vi "TDC_DAQV30_Paralled_muon.vi"(7 "address":string[](array[string])=["192.168.10.20"], 8 "error in (no error)":errorcluster, 9 "stop":bool, 10 "save data":bool=TRUE, 11 "SMA mode":bool=TRUE) -> (0 "error out 3":errorcluster, 2 "csv path":path=path "G:/tdc/2017/data/test_20250313_082908.csv", 3 "rate":dbl)   [LabVIEW 2017]
uses:
  gloabal.vi
  <vilib>/Utility/file.llb/Write Delimited Spreadsheet (DBL).vi
  <vilib>/Utility/file.llb/Write Delimited Spreadsheet (I64).vi
panel:
  out "pmt trigger rate":u32[](array[numeric])
  out "event":u32[](array[numeric])
  in  "calib_file":path=path "G:/tdc/2017/data/test_20250313_032748_codeDensity.csv" caption="文件路径 （空时为对话框）"
  in  "use_calib_file":bool
  out "cal 3":u32[](graph)=[0, 0, 0, 0, 0, 0, 0, 0, 0, 0, 0, 0, 0, 0, 0, 0, 0, 0, 0, 0, 0, 0, 0, 0, 0, 0, 0, 0, 0, 0, 0, 0, 0, 0, 0, 0, 0, 0, 0, 0, 0, 0, 0, 0, 0, 0, 0, 0, 0, 0, 0, 0, 0, 0, 0, 0, 0, 0, 0, 0, 0, 0, 0, 0, 0, 0, 0, 0, 0, 0, 0, 0, 0, 0, 0, 0, 0, 0, 0, 0, 0, 0, 0, 0, 0, 0, 0, 0, 0, 0, 0, 0, 0, 0, 0, 0, 0, 0, 0, 0, 0, 0, 0, 0, 0, 0, 0, 0, 0, 0, 0, 0, 0, 0, 0, 0, 0, 0, 0, 0, 0, 0, 0, 0, 0, 0, 0, 0, 0, 0, 0, 0, 0, 0, 0, 0, 0, 0, 0, 0, 0, 0, 0, 0, 0, 0, 0, 0, 0, 0, 0, 0, 0, 0, 0, 0, 0, 0, 0, 0, 0, 0, 0, 0, 0, 15, 3, 1, 14, 3, 31, 20, 16, 6, 1, 18, 12, 4, 29, 10, 8, 29, 2, 14, 4, 25, 7, 24, 4, 0, 1, 5, 8, 18, 22, 0, 4, 5, 0, 12, 9, 9, 20, 21, 4, 10, 13, 5, 21, 13, 14, 2, 6, 13, 1, 3, 5, 10, 20, 2, 3, 4, 3, 4, 2, 20, 13, 2, 5, 1, 3, 12, 4, 1, 14, 7, 5, 4, 1, 10, 2, 21, 14, 2, 5, 10, 4, 0, 11, 19, 6, 4, 1, 37, 1, 4, 2, 1, 10, 13, 4, 8, 10, 6, 9, 2, 0, 6, 8, 12, 3, 21, 5, 7, 8, 2, 3, 7, 17, 6, 5, 6, 4, 6, 0, 2, 1, 3, 10, 33, 7, 2, 6, 3, 7, 3, 2, 0, 12, 10, 11, 13, 13, 7, 3, 9, 6, 16, 0, 13, 5, 6, 3, 0, 5, 5, 7, 1, 10, 7, 13, 14, 5, 1, 12, 7, 1, 10, 2, 1, 14, 18, 13, 11, 4, 6, 9, 22, 11, 9, 2, 2, 8, 14, 4, 4, 6, 12, 13, 3, 9, 5, 5, 1, 5, 11, 18, 3, 0, 5, 4, 6, 7, 6, 1, 13, 5, 1, 2, 2, 1, 4, 12, 7, 3, 2, 3, 9, 11, 1, 20, 3, 4, 5, 5, 3, 5, 8, 5, 3, 26, 14, 6, 1, 3, 12, 12, 4, 23, 10, 3, 4, 4, 10, 3, 5, 4, 2, 14, 5, 15, 20, 1, 5, 1, 20, 6, 1, 3, 13, 21, 12, 7, 4, 1, 5, 30, 11, 2, 4, 0, 12, 7, 10, 3, 2, 25, 6, 1, 3, 6, 3, 8, 37, 4, 6, 2, 2, 4, 3, 5, 6, 13, 6, 9, 22, 1, 3, 7, 7, 4, 8, 33, 2, 1, 15, 3, 8, 23, 21, 2, 2, 27, 13, 3, 5, 10, 4, 18, 5, 5, 8, 0, 1, 8, 12, 4, 3, 0, 4, 8, 4, 7, 4, 2, 11, 13, 3, 0, 7, 5, 3, 4, 8, 4, 20, 2, 13, 4, 8, 6, 17, 4, 2, 1, 15, 2, 15, 5, 19, 0, 4, 15, 4, 16, 11, 1, 16, 4, 6, 6, 5, 7, 3, 9, 15, 3, 6, 3, 13, 5, 7, 3, 27, 2, 0, 21, 1, 4, 1, 4, 5, 3, 10, 7, 3, 6, 4, 18, 21, 7, 6, 7, 7, 12, 6, 9, 8, 11, 12, 13, 2, 2, 5, 4, 7, 52, 3, 5, 8, 7, 10, 4, 4, 6, 5, 18, 0, 3, 6, 1, 9, 5, 19, 13, 24, 12, 4, 4, 15, 6, 41, 3, 8, 5, 17, 26, 8, 7, 20, 2, 5, 12, 10, 10, 12, 9, 17, 6, 3, 1, 5, 3, 7, 8, 4, 10, 5, 10, 7, 1, 2, 14, 7, 25, 3, 0, 0, 0, 5, 21, 8, 14, 4, 10, 2, 3, 2, 4, 8, 12, 3, 6, 8, 3, 4, 3, 20, 5, 6, 7, 8, 11, 2, 8, 6, 5, 15, 17, 10, 10, 3, 3, 9, 18, 7, 7, 3, 5, 5, 5, 2, 2, 2, 4, 1, 0, 42, 3, 14, 4, 3, 5, 2, 7, 4, 2, 7, 5, 22, 4, 3, 17, 3, 5, 8, 19, 7, 5, 0, 3, 4, 10, 1, 8, 2, 2, 13, 23, 4, 9, 5, 0, 0, 0, 27, 2, 16, 11, 15, 3, 0, 18, 2, 8, 29, 19, 6, 7, 2, 6, 12, 1, 13, 2, 7, 5, 11, 8, 5, 6, 6, 19, 2, 4, 0, 7, 22, 13, 3, 7, 3, 8, 11, 0, 3, 26, 6, 5, 5, 6, 4, 10, 17, 16, 4, 3, 4, 3, 4, 21, 8, 10, 10, 7, 0, 9, 9, 2, 10, 10, 2, 9, 9, 4, 14, 5, 5, 4, 18, 6, 3, 0, 4, 1, 20, 2, 33, 4, 1, 2, 1, 20, 6, 3, 11, 10, 2, 1, 13, 9, 6, 1, 0, 0, 0, 0, 0, 0, 0, 0, 0, 0, 0, 0, 0, 0, 0, 0, 0, 0, 0, 0, 0, 0, 0, 0, 0, 0, 0, 0, 0, 0, 0, 0, 0, 0, 0, 0, 0, 0, 0, 0, 0, 0, 0, 0, 0, 0, 0, 0, 0, 0, 0, 0, 0, 0, 0, 0, 0, 0, 0, 0, 0, 0, 0, 0, 0, 0, 0, 0, 0, 0, 0, 0, 0, 0, 0, 0, 0, 0, 0, 0, 0, 0, 0, 0, 0, 0, 0, 0, 0, 0, 0, 0, 0, 0, 0, 0, 0, 0, 0, 0, 0, 0, 0, 0, 0, 0, 0, 0, 0, 0, 0, 0, 0, 0, 0, 0, 0, 0, 0, 0, 0, 0, 0, 0, 0, 0, 0, 0, 0, 0, 0, 0, 0, 0, 0, 0, 0, 0, 0, 0, 0, 0, 0, 0, 0, 0, 0, 0, 0, 0, 0, 0, 0, 0, 0, 0, 0, 0, 0, 0, 0, 0, 0, 0, 0, 0, 0, 0, 0, 0, 0, 0, 0, 0, 0, 0, 0, 0, 0, 0, 0, 0, 0, 0, 0, 0, 0, 0, 0, 0, 0, 0, 0, 0, 0, 0, 0, 0, 0, 0, 0, 0, 0, 0, 0, 0, 0, 0, 0, 0, 0, 0, 0, 0, 0, 0, 0, 0, 0, 0, 0, 0, 0, 0, 0, 0, 0, 0, 0, 0, 0, 0, 0, 0, 0, 0, 0, 0, 0, 0, 0, 0, 0, 0, 0, 0, 0, 0, 0, 0, 0, 0, 0, 0, 0, 0, 0, 0, 0, 0, 0, 0, 0, 0, 0, 0, 0, 0, 0, 0, 0, 0, 0, 0, 0, 0, 0, 0, 0, 0, 0, 0, 0, 0, 0, 0, 0, 0, 0, 0, 0, 0, 0, 0, 0, 0, 0, 0, 0, 0, 0, 0, 0, 0, 0, 0, 0, 0, 0, 0, 0, 0, 0, 0, 0, 0, 0, 0, 0, 0, 0, 0, 0, 0, 0, 0, 0, 0, 0, 0, 0, 0, 0, 0, 0, 0, 0, 0, 0, 0, 0, 0, 0, 0, 0, 0, 0, 0, 0, 0, 0, 0, 0, 0, 0, 0, 0, 0, 0, 0, 0, 0, 0, 0, 0, 0, 0, 0, 0, 0, 0, 0, 0, 0, 0, 0, 0, 0, 0, 0, 0, 0, 0, 0, 0, 0, 0, 0, 0, 0, 0, 0, 0, 0, 0, 0, 0, 0, 0, 0, 0, 0, 0, 0, 0, 0, 0, 0, 0, 0, 0, 0, 0, 0, 0, 0, 0, 0, 0, 0, 0, 0, 0, 0, 0, 0, 0, 0, 0, 0, 0, 0, 0, 0, 0, 0, 0, 0, 0, 0, 0, 0, 0, 0, 0, 0, 0, 0, 0, 0, 0, 0, 0, 0, 0, 0, 0, 0, 0, 0, 0, 0, 0, 0, 0, 0, 0, 0, 0, 0, 0, 0, 0, 0, 0, 0, 0, 0, 0, 0, 0, 0, 0, 0, 0, 0, 0, 0, 0, 0, 0, 0, 0, 0, 0, 0, 0, 0, 0, 0, 0, 0, 0, 0, 0, 0, 0, 0, 0, 0, 0, 0, 0, 0, 0, 0, 0, 0, 0, 0, 0, 0, 0, 0, 0, 0, 0, 0, 0, 0, 0, 0, 0, 0, 0, 0, 0, 0, 0, 0, 0, 0, 0, 0, 0, 0, 0, 0, 0, 0, 0, 0, 0, 0, 0, 0, 0, 0, 0, 0, 0, 0, 0, 0, 0, 0, 0, 0, 0, 0, 0, 0, 0, 0, 0, 0, 0, 0, 0, 0, 0, 0, 0, 0, 0, 0, 0, 0, 0, 0, 0, 0, 0, 0, 0, 0, 0, 0, 0, 0, 0, 0, 0, 0, 0, 0, 0, 0, 0, 0, 0, 0, 0, 0, 0, 0, 0, 0, 0, 0, 0, 0, 0, 0, 0, 0, 0, 0, 0, 0, 0, 0, 0, 0, 0, 0, 0, 0, 0, 0, 0, 0, 0, 0, 0, 0, 0, 0, 0, 0, 0, 0, 0, 0, 0, 0, 0, 0, 0, 0, 0, 0, 0, 0, 0, 0, 0, 0, 0, 0, 0, 0, 0, 0, 0, 0, 0, 0, 0, 0, 0, 0, 0, 0, 0, 0, 0, 0, 0, 0, 0, 0, 0, 0, 0, 0, 0, 0, 0, 0, 0, 0, 0, 0, 0, 0, 0, 0, 0, 0, 0, 0, 0, 0, 0, 0, 0, 0, 0, 0, 0, 0, 0, 0, 0, 0, 0, 0, 0, 0, 0, 0, 0, 0, 0, 0, 0, 0, 0, 0, 0, 0, 0, 0, 0, 0, 0, 0, 0, 0, 0, 0, 0, 0, 0, 0, 0, 0, 0, 0, 0, 0, 0, 0, 0, 0, 0, 0, 0, 0, 0, 0, 0, 0, 0, 0, 0, 0, 0, 0, 0, 0, 0, 0, 0, 0, 0, 0, 0, 0, 0, 0, 0, 0, 0, 0, 0, 0, 0, 0, 0, 0, 0, 0, 0, 0, 0, 0, 0, 0, 0, 0, 0, 0, 0, 0, 0, 0, 0, 0, 0, 0, 0, 0, 0, 0, 0, 0, 0, 0, 0, 0, 0, 0, 0, 0, 0, 0, 0, 0, 0, 0, 0, 0, 0, 0, 0, 0, 0, 0, 0, 0, 0, 0, 0, 0, 0, 0, 0, 0, 0, 0, 0, 0, 0, 0, 0, 0, 0, 0, 0, 0, 0, 0, 0, 0, 0, 0, 0, 0, 0, 0, 0, 0, 0, 0, 0, 0, 0, 0, 0, 0, 0, 0, 0, 0, 0, 0, 0, 0, 0, 0, 0, 0, 0, 0, 0, 0, 0, 0, 0, 0, 0, 0, 0, 0, 0, 0, 0, 0, 0, 0, 0, 0, 0, 0, 0, 0, 0, 0, 0, 0, 0, 0, 0, 0, 0, 0, 0, 0, 0, 0, 0, 0, 0, 0, 0, 0, 0, 0, 0, 0, 0, 0, 0, 0, 0, 0, 0, 0, 0, 0, 0, 0, 0, 0, 0, 0, 0, 0, 0, 0, 0, 0, 0, 0, 0, 0, 0, 0, 0, 0, 0, 0, 0, 0, 0, 0, 0, 0, 0, 0, 0, 0, 0, 0, 0, 0, 0, 0, 0, 0, 0, 0, 0, 0, 0, 0, 0, 0, 0, 0, 0, 0, 0, 0, 0, 0, 0, 0, 0, 0, 0, 0, 0, 0, 0, 0, 0, 0, 0, 0, 0, 0, 0, 0, 0, 0, 0, 0, 0, 0, 0, 0, 0, 0, 0, 0, 0, 0, 0, 0, 0, 0, 0, 0, 0, 0, 0, 0, 0, 0, 0, 0, 0, 0, 0, 0, 0, 0, 0, 0, 0, 0, 0, 0, 0, 0, 0, 0, 0, 0, 0, 0, 0, 0, 0, 0, 0, 0, 0, 0, 0, 0, 0, 0, 0, 0, 0, 0, 0, 0, 0, 0, 0, 0, 0, 0, 0, 0, 0, 0, 0, 0, 0, 0, 0, 0, 0, 0, 0, 0, 0, 0, 0, 0, 0, 0, 0, 0, 0, 0, 0, 0, 0, 0, 0, 0, 0, 0, 0, 0, 0, 0, 0, 0, 0, 0, 0, 0, 0, 0, 0, 0, 0, 0, 0, 0, 0, 0, 0, 0, 0, 0, 0, 0, 0, 0, 0, 0, 0, 0, 0, 0, 0, 0, 0, 0, 0, 0, 0, 0, 0, 0, 0, 0, 0, 0, 0, 0, 0, 0, 0, 0, 0, 0, 0, 0, 0, 0, 0, 0, 0, 0, 0, 0, 0, 0, 0, 0, 0, 0, 0, 0, 0, 0, 0, 0, 0, 0, 0, 0, 0, 0, 0]
  out "second stamp":u64=57608
  in  "coarse counter width":u16(ring) items=["29", "48"]
  out "name (unnamed)":string
  out "error out 5":errorcluster
  in  "timeout":dbl=30000.0
  out "DAC":dbl=8094.0
  out "Out":u8=3 format="%.0x"
  out "fine 4":u64=133527214080 format="%x"
  out "coarse":u64=65198835 format="%x"
  in  "gps":bool
  out "Year":string="2025"
  in  "factor":i32=128
  in  "displayCR":bool=TRUE
  in  "Counter Setting":dbl=100000.0 format="%#_13g"
  in  "replace dat":bool
  in  "append csv":bool=TRUE
  out "element":string
  out "fine":u64=593 format="%x"
  in  "UDP Config":bool=TRUE
  in  "data  path":path=path "G:/tdc/2017/data"
  out "cal 2":u64[](graph)
  in  "Thresholds (mV)":dbl[](array[numeric])=[580.0, 580.0, 580.0, 580.0, 600.0, 600.0, 600.0, 600.0, 580.0, 580.0, 600.0, 600.0, 600.0, 600.0, 600.0, 600.0, 580.0, 580.0, 600.0, 600.0, 600.0, 600.0, 600.0, 600.0, 580.0, 580.0, 600.0, 600.0, 600.0, 600.0, 600.0, 600.0, 600.0, 600.0, 600.0, 600.0, 600.0, 600.0, 600.0, 600.0, 600.0, 600.0, 600.0, 600.0, 600.0, 600.0, 600.0, 600.0, 600.0, 600.0, 600.0, 600.0, 600.0, 600.0, 600.0, 600.0, 600.0, 600.0, 600.0, 600.0, 600.0, 600.0, 600.0, 600.0]
  out "error out 2":errorcluster
  in  "display":bool=TRUE
  in  "Thresholds":dbl=-0.03
  in  "one key for threshold":bool=TRUE
  in  "RST":bool
  in  "通道数量":i32=128
  out "Cal Table":u32[](array[numeric])
  in  "channel for cal":i32=3
  out "channel number":u64
  out "Calibration Counter":i32=100000
  out "Event index":i32=97959
  out "cal":i64[](graph)
  out "error out":errorcluster
  out "appended path":path=path "G:/tdc/2017/data/test_20250313_082908.dat"
  in  "filename":string="test"
  in  "Events":i32=110000 min=1
  in  "timeout (ms)":i32=10000
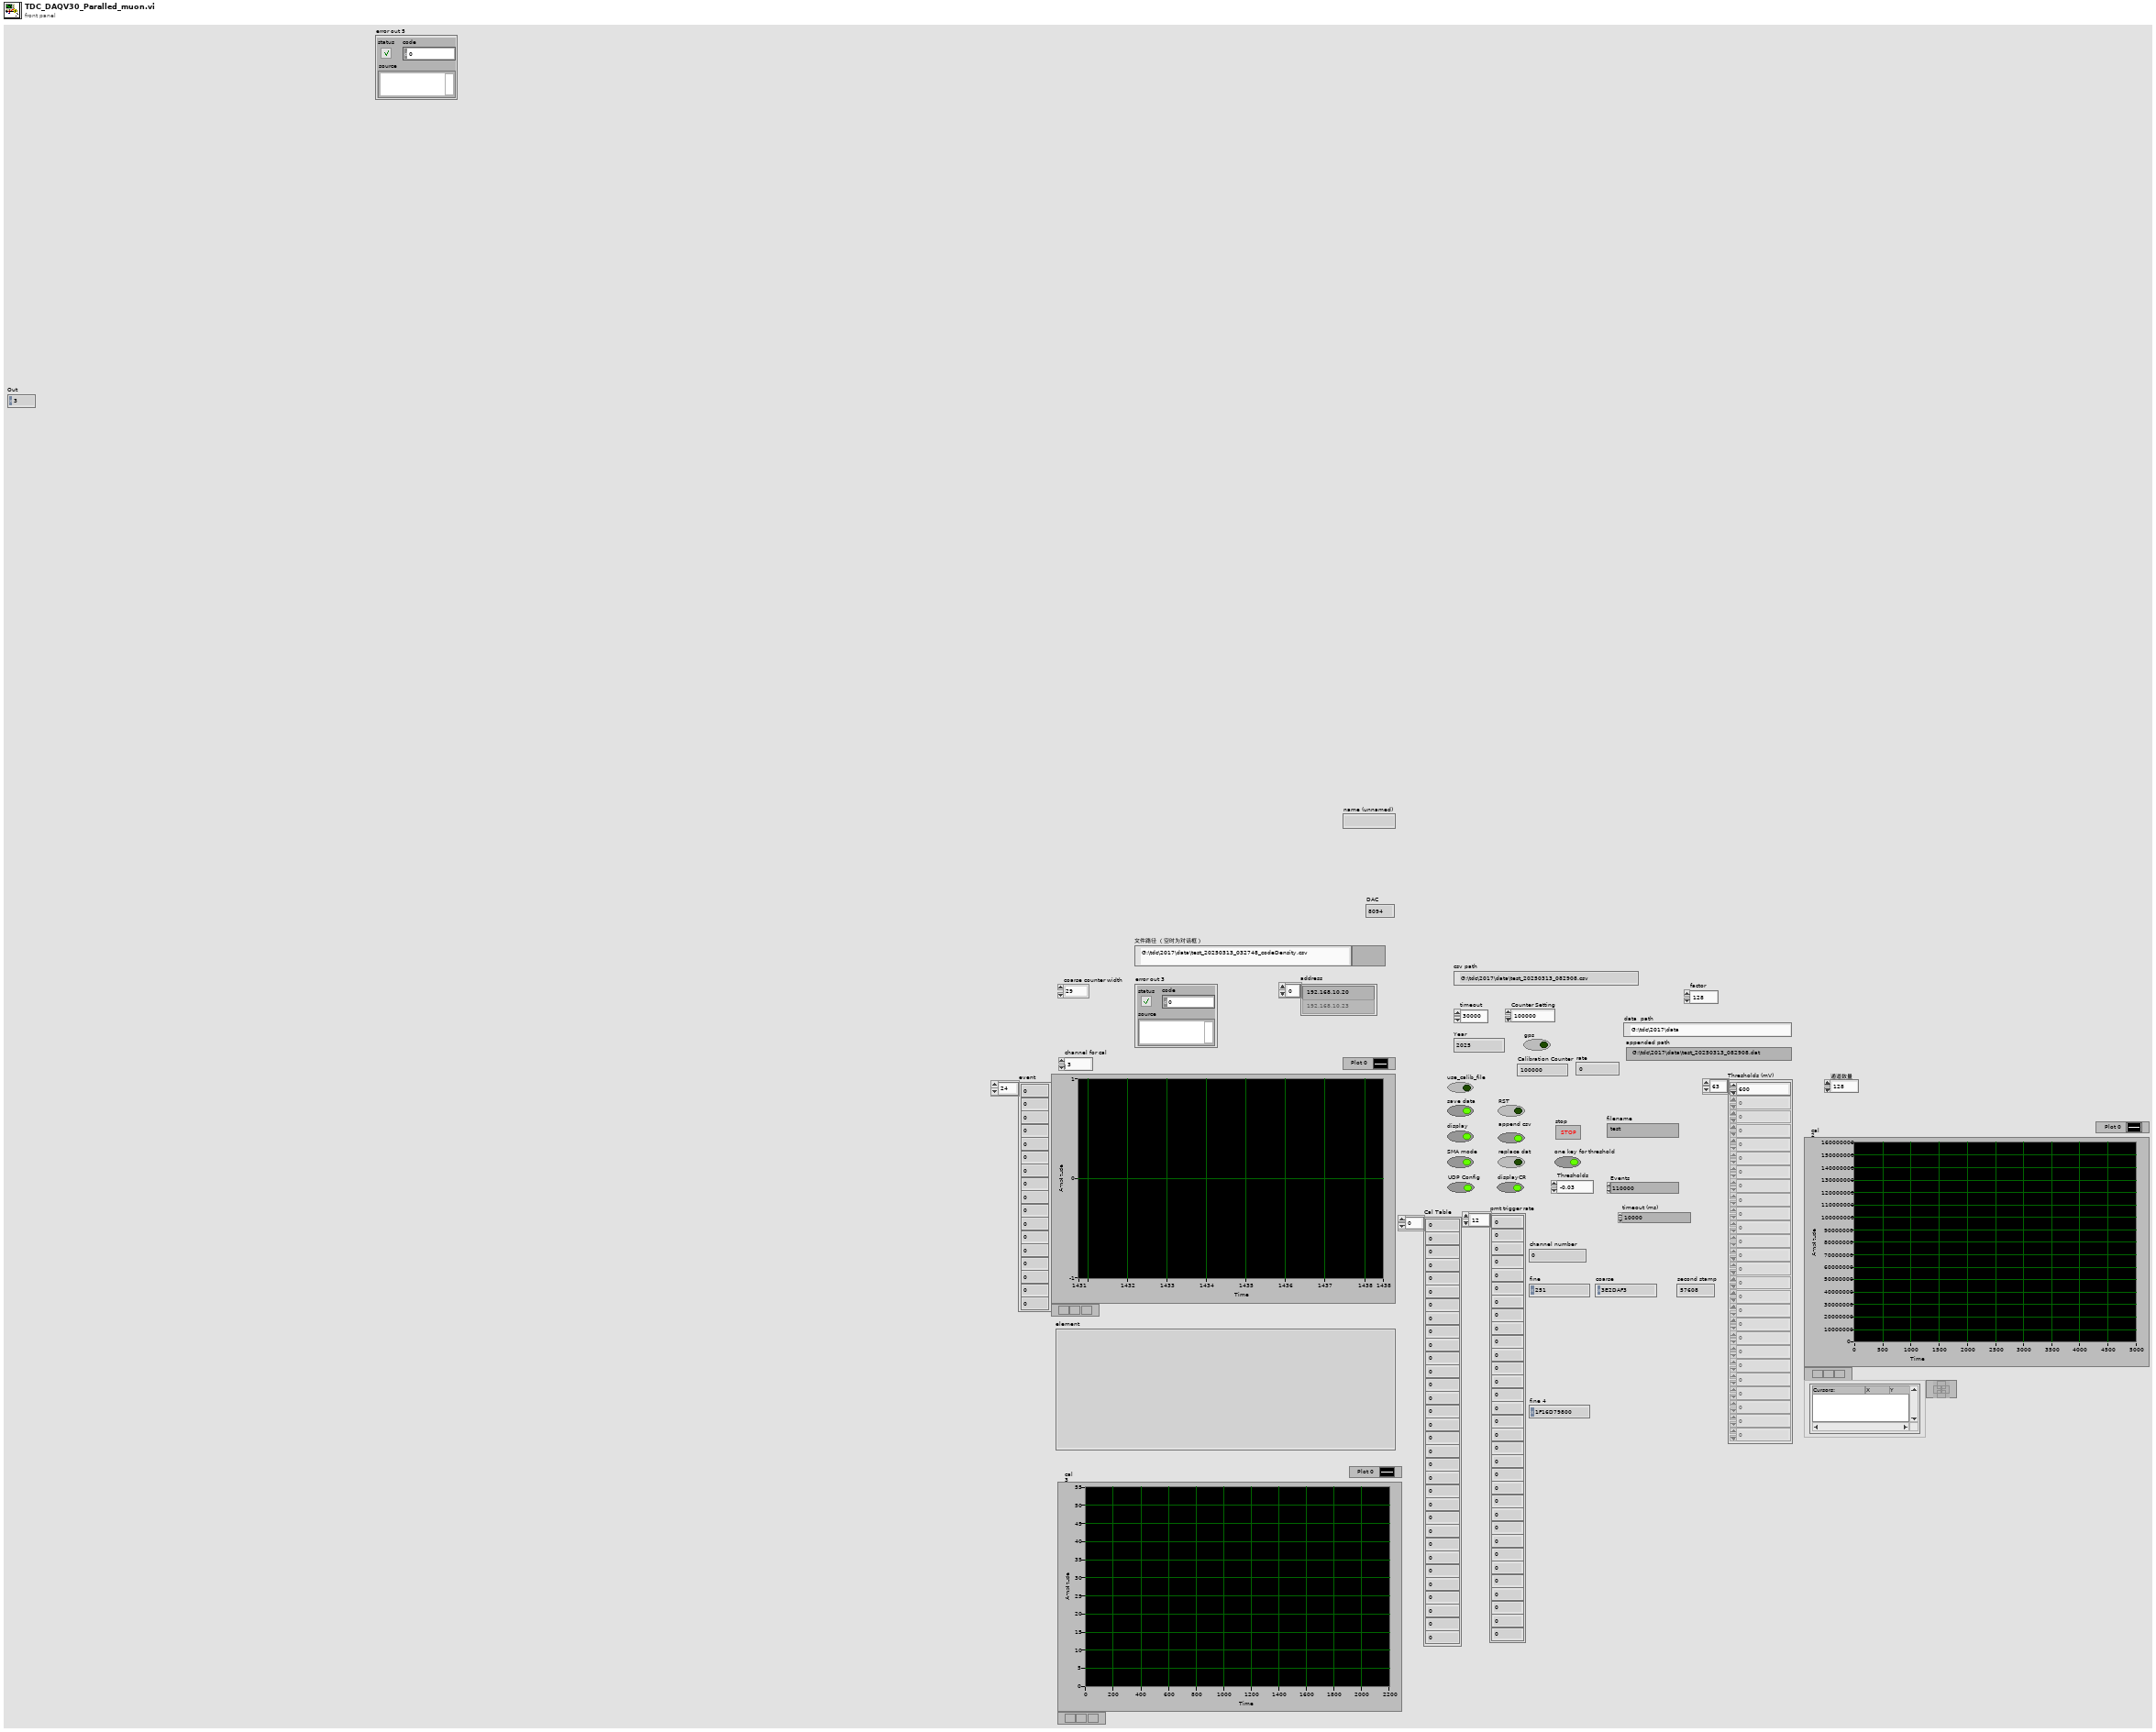
[diagram p1: front panel]
types:
  T1 = enum16{"open", "replace", "create", "open or create", "replace or create", "replace or create with confirmation"}
  T2 = enum16{"big-endian, network order", "native, host order", "little-endian"}
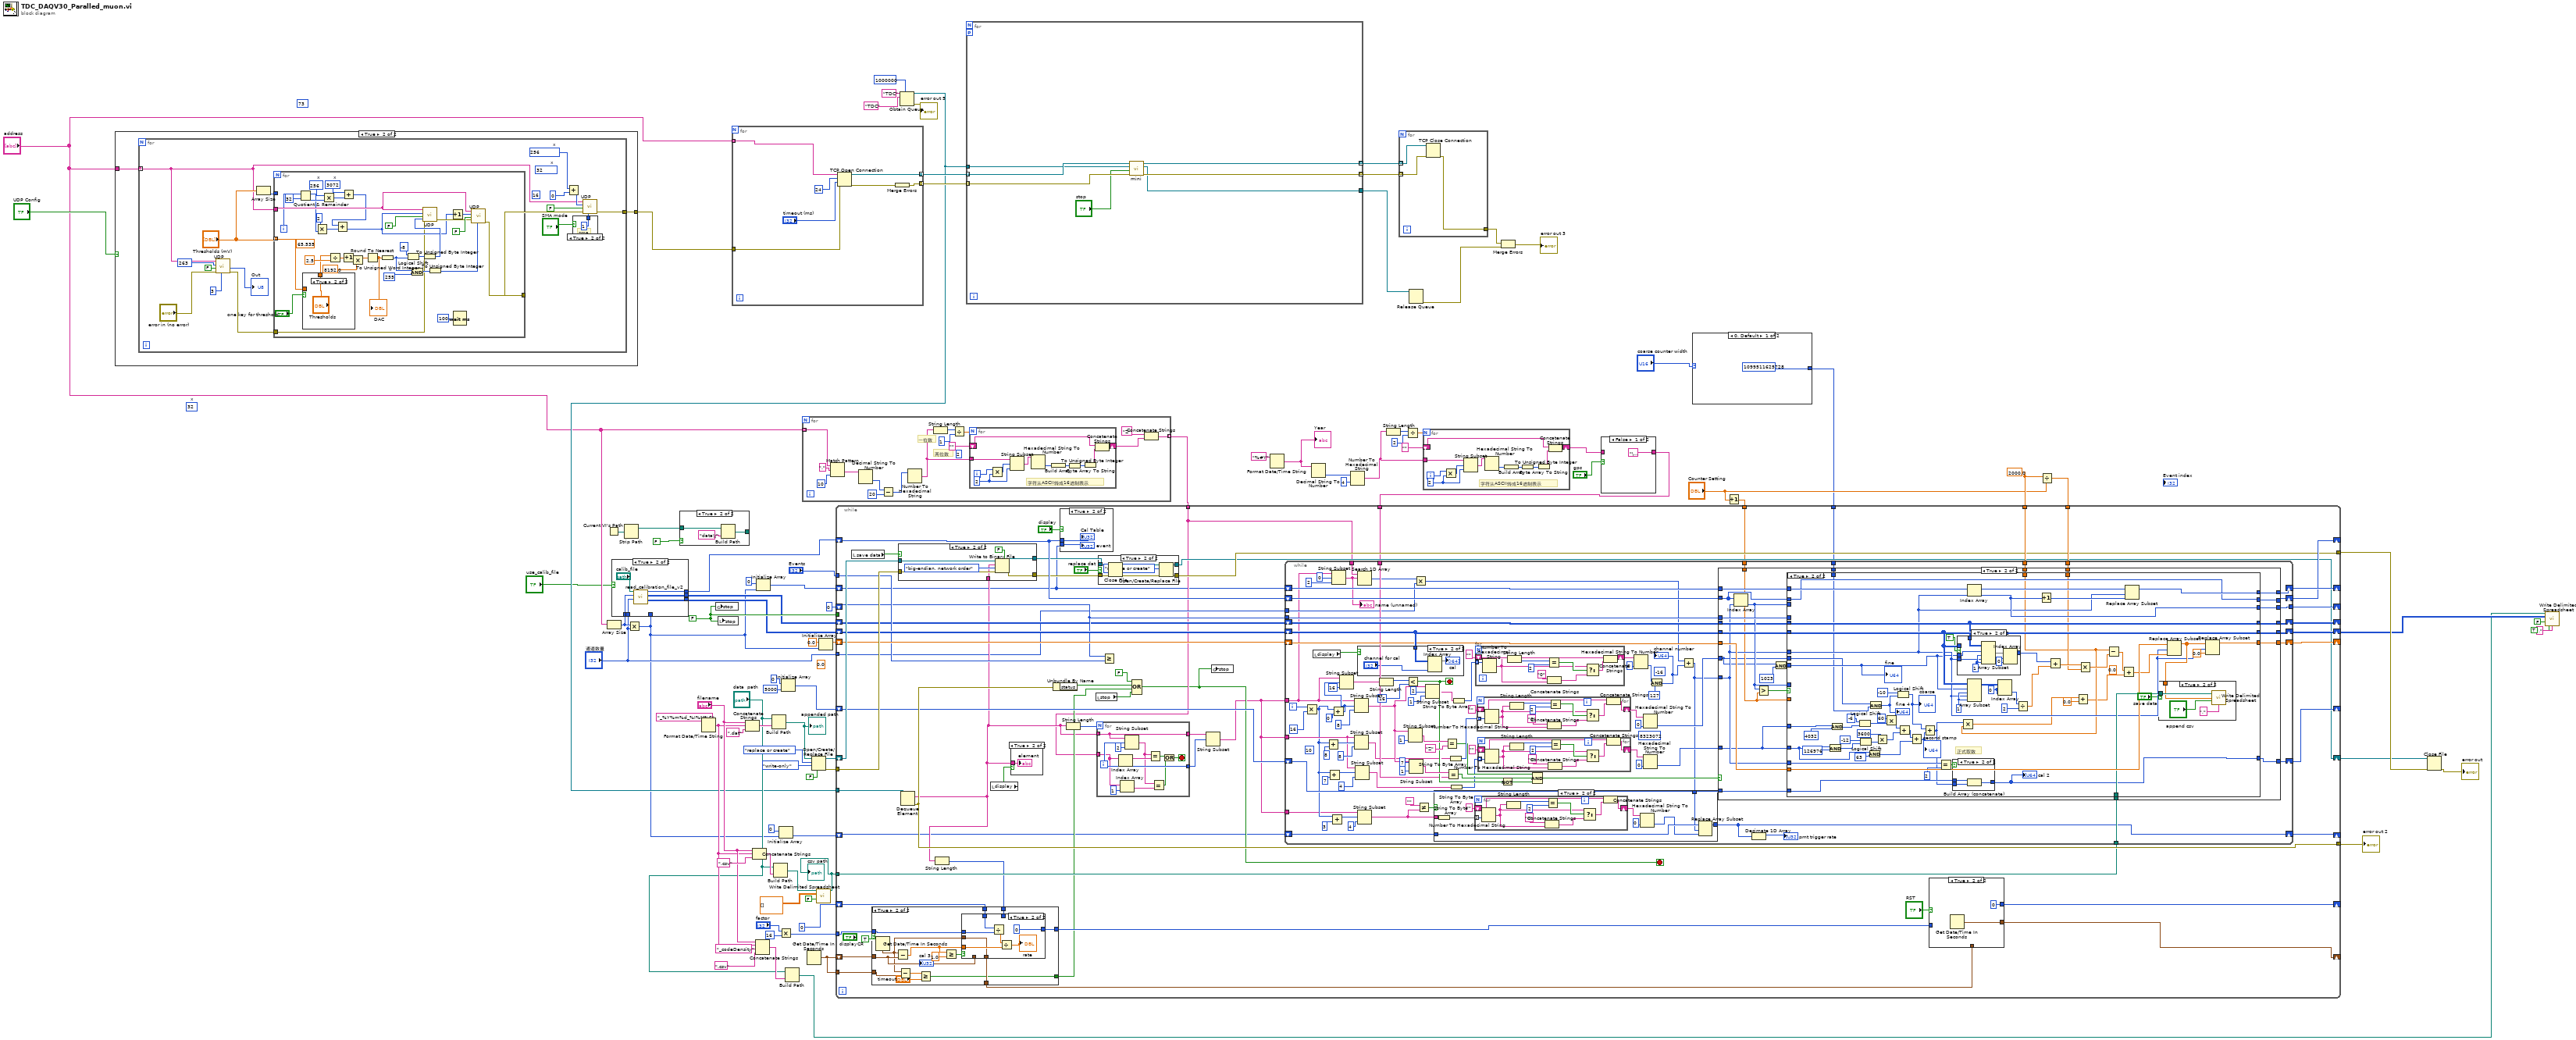
[diagram p0: block diagram]
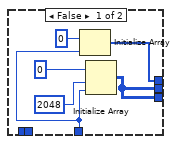
[diagram p2: hidden frame]
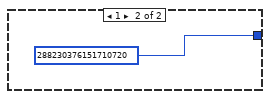
[diagram p3: hidden frame]
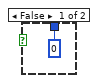
[diagram p6: hidden frame]
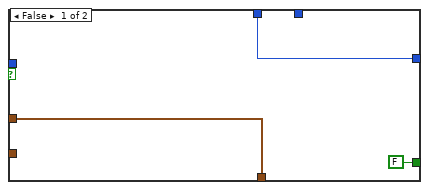
[diagram p12: hidden frame]
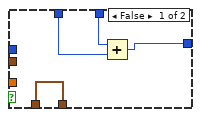
[diagram p13: hidden frame]
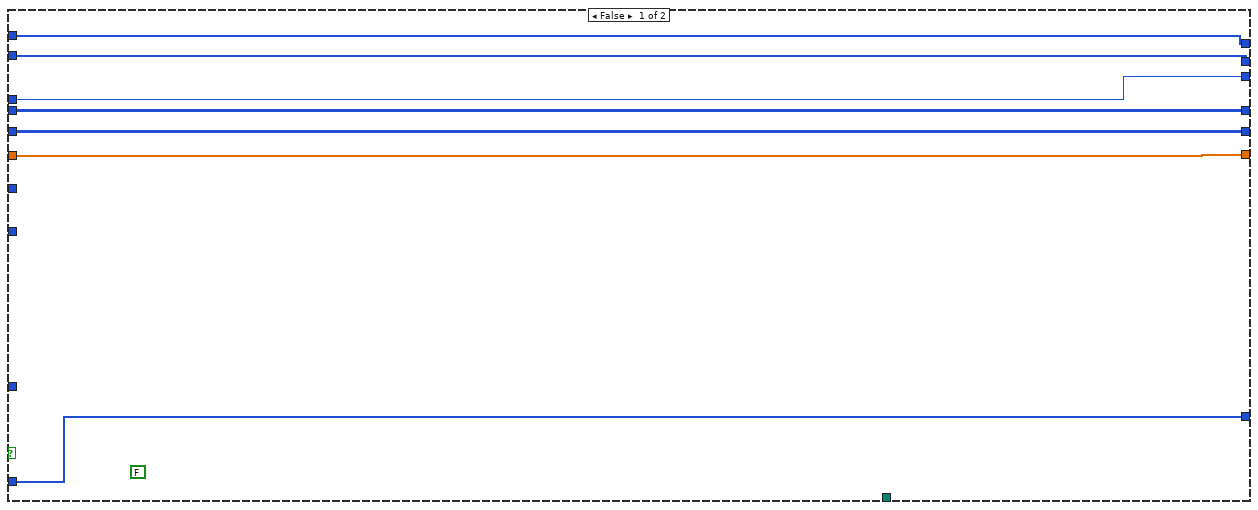
[diagram p18: hidden frame]
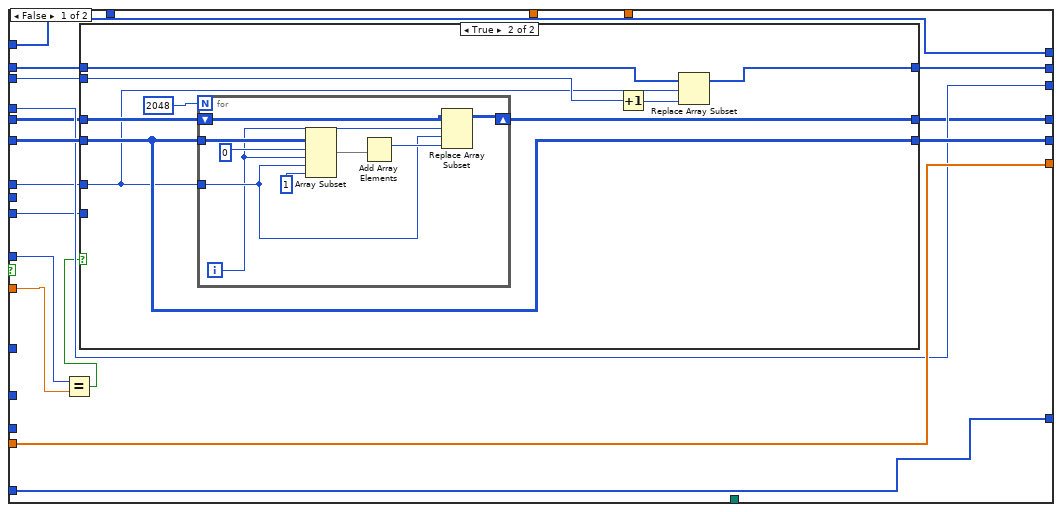
[diagram p19: hidden frame]
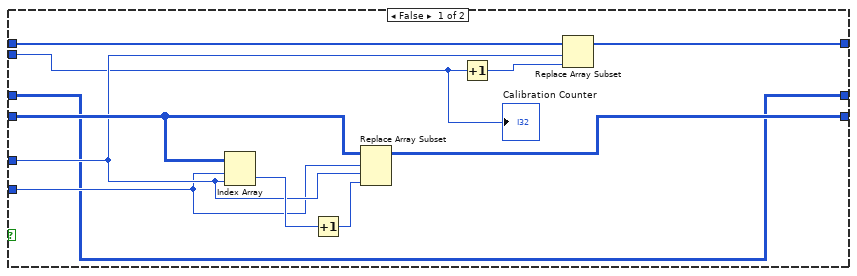
[diagram p20: hidden frame]
diagram:
  (unwired) u32 73 ("Address")
  w51 = 2000.0 ("x")
  (unwired) u16 32  # x
  w13 = FALSE ("stop")
  (unwired) 0.0
  n1 = case shown="True" "UDP Config" {
    tunnel: "address" -> [_ w93]
    tunnel: [_ w94] -> w18
    frame False {
    }
    frame True {
      n2 = for {
        tunnel: [w109] -> w94
        tunnel: w93 -> [w97] mode=indexing
        (unwired) u16 32  # x
        (unwired) u32 16 ("Address")
        w102 = u16 256  # x
        n3 = call "UDP.vi"("In"=u8 3, "error in (no error)"="error in (no error)", "Read (TRUE)"=FALSE, "Address"=u32 263, "IP address"=w97) -> ("error out"=w95:errorcluster, "Out"=→"Out":u8)  [unwired: 3 in, 1 out]
        n4 = Array Size(array="Thresholds (mV)") -> (size(s)=w106:i32)
        n5 = for {
          tunnel: w97 -> [w143]
          tunnel: "Thresholds (mV)" -> [w130] mode=indexing
          tunnel: [w133] -> w110
          tunnel: w106 -> [_]
          tunnel: w95 -> [w117]
          i -> [w125]
          (unwired) 65.535 ("y")
          w126 = u16 3072  # x
          w127 = u16 256  # x
          w139 = u16 255  # x
          n6 = Quotient & Remainder(x=w125, y=32) -> (x-y*floor(x/y)=w119:i32, floor(x/y)=w128:i32)
          n7 = case shown="True" "one key for threshold" {
            tunnel: [w149 "Thresholds"] -> w131
            tunnel: w130 -> [w149 _]
            frame False {
            }
            frame True {
            }
          }
          n8 = Multiply(x=2, y=w119) -> (x*y=w120:i32)
          n9 = Multiply(x=w127, y=w128) -> (x*y=w122:i32)
          n10 = Divide(x=w131, y=2.5) -> (x/y=w146:dbl)
          n11 = Increment(x=w146) -> (x+1=w116:dbl)
          n12 = Add(x=w126, y=w122) -> (x+y=w121:i32)
          n13 = Add(x=w121, y=w120) -> (x+y=w124:i32)
          n14 = Multiply(x=w116, y=8192.0) -> (x*y=w115:dbl)
          n15 = Round To Nearest(number=w115) -> (nearest integer value=w144:dbl)
          "DAC" <- w144
          n16 = To Unsigned Word Integer(number=w144) -> (unsigned 16bit integer=w135:u16)
          n17 = Logical Shift(y=i16 -8, x=w135) -> (x << y=w141:u16)
          n18 = And(x=w135, y=w139) -> (x .and. y?=w138:u16)
          n19 = To Unsigned Byte Integer(number=w141) -> (unsigned 8bit integer=w140:u8)
          n20 = call "UDP.vi"("In"=w140, "error in (no error)"=w117, "Read (TRUE)"=FALSE, "Address"=w124, "IP address"=w143) -> ("error out"=w134:errorcluster)  [unwired: 3 in, 2 out]
          n21 = To Unsigned Byte Integer(number=w138) -> (unsigned 8bit integer=w137:u8)
          n22 = Increment(x=w124) -> (x+1=w123:i32)
          n23 = Wait (ms)(milliseconds to wait=u32 100) -> ()  [unwired: 1 out]
          n24 = call "UDP.vi"("In"=w137, "error in (no error)"=w134, "Read (TRUE)"=FALSE, "Address"=w123, "IP address"=w143) -> ("error out"=w133:errorcluster)  [unwired: 3 in, 2 out]
        }
        n25 = Add(x=w102, y=u32 0 ("Address")) -> (x+y=w103:u32)
        n26 = case shown="True" "SMA mode" {
          tunnel: [u8 0 ("In") u8 1 ("In")] -> w108
          frame False {
          }
          frame True {
            # "sma"
          }
        }
        n27 = call "UDP.vi"("In"=w108, "error in (no error)"=w110, "Read (TRUE)"=FALSE, "Address"=w103, "IP address"=w97) -> ("error out"=w109:errorcluster)  [unwired: 3 in, 2 out]
      }
    }
  }
  n28 = Current VI's Path() -> (path=w87:path)
  n29 = Array Size(array="address") -> (size(s)=w5:i32)
  n30 = Strip Path(path=w87) -> (stripped path=w86:path)  [unwired: 1 out]
  n31 = Multiply(x=w5, y="通道数量") -> (x*y=w2:i32)
  n32 = case shown="True" "use_calib_file" {
    tunnel: w2 -> [w154 _]
    tunnel: [w151 w162] -> w8
    tunnel: [w151 w161] -> w7
    tunnel: [w152 w160] -> w6
    tunnel: w5 -> [_ w159]
    tunnel: "通道数量" -> [_ w158]
    frame False {
      n33 = Initialize Array(u32 0 ("element"), w154) -> (w152:u32[])
      n34 = Initialize Array(u32 0 ("element"), 2048 ("dimension size"), w154) -> (w151:u32[][])
    }
    frame True {
      n35 = call "read_calibration_file_v2.vi"("通道数量"=w158, "板子数量"=w159, "file path (dialog if empty)"="calib_file") -> ("code_density"=w162:i64[][], "accumulation"=w161:u32[][], "Cal Table"=w160:u32[])  [unwired: 5 in, 1 out]
    }
  }
  n36 = case shown="True" FALSE {
    tunnel: w86 -> [w163 w165]
    tunnel: [w163 w164] -> _
    frame False {
    }
    frame True {
      n37 = Build Path(base path=w165, name or relative path="data\\") -> (appended path=w164:path)
    }
  }
  n38 = Format Date/Time String(time format string (%c)="_%Y%m%d_%I%M%S") -> (date/time string=w68:string)  [unwired: 2 in]
  n39 = global write "gloabal.vi" "stop"(w13) -> ()
  n40 = local write "stop"(w13) -> ()
  n41 = for {
    tunnel: "address" -> [w172] mode=indexing
    tunnel: [w171] -> w28 mode=indexing
    tunnel: [w169] -> w27 mode=indexing
    tunnel: w18 -> [w168]
    n42 = TCP Open Connection(address=w172, remote port or service name=u16 24 ("port"), timeout ms (60000)="timeout (ms)", error in (no error)=w168) -> (connection ID=w171:refnum<k5>, error out=w170:errorcluster)  [unwired: 1 in]
    n43 = Merge Errors(w170) -> (w169:errorcluster)
  }
  n44 = Concatenate Strings("filename", w68, ".dat") -> (w85:string)
  n45 = Concatenate Strings("filename", w68, ".csv") -> (w75:string)
  n46 = Concatenate Strings("filename", w68, "_codeDensity" ("string"), ".csv") -> (w65:string)
  n47 = Initialize Array(u32 0 ("element"), w2) -> (w74:u32[])
  n48 = Build Path(base path="data  path", name or relative path=w85) -> (appended path=w84:path)
  "appended path" <- w84
  n49 = Build Path(base path="data  path", name or relative path=w75) -> (appended path=w72:path)
  n50 = Initialize Array(u32 0 ("element"), w2) -> (w1:u32[])
  n51 = Multiply(x="factor", y=16) -> (x*y=w44:i32)
  n52 = Initialize Array(u32 0 ("element"), 5000 ("dimension size")) -> (w56:u32[])
  n53 = Build Path(base path="data  path", name or relative path=w65) -> (appended path=w62:path)
  n54 = for {
    tunnel: [w175] -> w30 mode=indexing
    tunnel: "address" -> [w174] mode=indexing
    (unwired) 2 ("y")
    # "一位数"
    # "两位数"
    n55 = Match Pattern(string=w174, regular expression="." ("search string"), offset (0)=10) -> (after substring=w181:string)  [unwired: 3 out]
    n56 = Decimal String To Number(string=w181) -> (number=w178:i32)  [unwired: 2 in, 1 out]
    n57 = Subtract(x=w178, y=20) -> (x-y=w177:i32)
    n58 = Number To Hexadecimal String(2:w177) -> (0:w180:string)  [unwired: 1 in]
    n59 = String Length(string=w180) -> (length=w186:i32)
    n60 = Divide(x=w186, y=1) -> (x/y=w187:dbl)
    n61 = for {
      N: w187 -> [_]
      shift-right: [w199] -> w176
      shift-left: "" ("format string") -> [w198]
      tunnel: w180 -> [w189]
      i -> [w197]
      w191 = 2 ("y")
      # "字符从ASCII转成16进制表示"
      n62 = Multiply(x=w197, y=w191) -> (x*y=w190:i32)
      n63 = String Subset(string=w189, offset (0)=w190, length (rest)=w191) -> (substring=w192:string)
      n64 = Hexadecimal String To Number(string=w192) -> (number=w196:u32)  [unwired: 2 in, 1 out]
      n65 = Build Array(w196) -> (w195:u32[])
      n66 = To Unsigned Byte Integer(number=w195) -> (unsigned 8bit integer=w194:u8[])
      n67 = Byte Array To String(unsigned byte array=w194) -> (string=w193:string)
      n68 = Concatenate Strings(w198, w193) -> (w199:string)
    }
    n69 = Concatenate Strings("Z", w176) -> (w175:string)
  }
  n70 = Get Date/Time In Seconds() -> (seconds since 1Jan1904=w29:timestamp)
  n71 = Open/Create/Replace File(file path (use dialog)=w84, operation (0:open)=T1."replace or create", access (0:read/write)=enum16{"read/write", "read-only", "write-only"}."write-only", disable buffering (F)=FALSE) -> (refnum out=w89:refnum<file>, error out=w88:errorcluster)  [unwired: 2 in, 1 out]
  n72 = call-poly <vilib>:"Write Delimited Spreadsheet.vi"("file path (dialog if empty)"=w72, "2D data"=dbl[][] [], "append to file? (new file:F)"=FALSE) -> ("new file path (Not A Path if cancelled)"=w12:path)  [unwired: 11 in, 1 out]
  "csv path" <- w12
  n73 = Initialize Array(0.0, w2) -> (w58:dbl[])
  n74 = Obtain Queue(max queue size (-1, unlimited)=1000000, name (unnamed)="TDC", element data type="TDC" ("name (unnamed)")) -> (queue out=w19:refnum<queue>, error out=→"error out 5":errorcluster)  [unwired: 2 in, 1 out]
  n75 = for {
    tunnel: w28 -> [w206] mode=indexing
    tunnel: w27 -> [w205] mode=indexing
    tunnel: [w204] -> w26 mode=indexing
    tunnel: [w203] -> w25 mode=indexing
    workers-P: _ -> [_]
    tunnel: w19 -> [w202]
    tunnel: [w201] -> w20
    n76 = call "mini.vi"("error in (no error)"=w205, "stop"="stop", "queue out 2"=w202, "connection ID 2"=w206) -> ("error out 3"=w203:errorcluster, "queue out"=w201:refnum<queue>, "connection ID"=w204:refnum<k5>)  [unwired: 5 in]
  }
  n77 = Format Date/Time String(time format string (%c)="%#Y") -> (date/time string=w41:string)  [unwired: 2 in]
  "Year" <- w41
  n78 = Decimal String To Number(string=w41) -> (number=w40:i32)  [unwired: 2 in, 1 out]
  n79 = Number To Hexadecimal String(1:i16 4 ("width (-)"), 2:w40) -> (0:w34:string)
  n80 = String Length(string=w34) -> (length=w36:i32)
  n81 = for {
    tunnel: w26 -> [w209] mode=indexing
    tunnel: w25 -> [w208] mode=indexing
    tunnel: [w207] -> w17
    n82 = TCP Close Connection(connection ID=w209, error in (no error)=w208) -> (error out=w207:errorcluster)  [unwired: 1 in, 1 out]
  }
  n83 = Divide(x=w36, y=2) -> (x/y=w37:dbl)
  n84 = Release Queue(queue=w20) -> (error out=w16:errorcluster)  [unwired: 2 in, 2 out]
  n85 = for {
    N: w37 -> [_]
    shift-right: [w220] -> w33
    shift-left: "" ("format string") -> [w219]
    tunnel: w34 -> [w210]
    i -> [w218]
    w212 = 2 ("y")
    # "字符从ASCII转成16进制表示"
    n86 = Multiply(x=w218, y=w212) -> (x*y=w211:i32)
    n87 = String Subset(string=w210, offset (0)=w211, length (rest)=w212) -> (substring=w213:string)
    n88 = Hexadecimal String To Number(string=w213) -> (number=w217:u32)  [unwired: 2 in, 1 out]
    n89 = Build Array(w217) -> (w216:u32[])
    n90 = To Unsigned Byte Integer(number=w216) -> (unsigned 8bit integer=w215:u8[])
    n91 = Byte Array To String(unsigned byte array=w215) -> (string=w214:string)
    n92 = Concatenate Strings(w219, w214) -> (w220:string)
  }
  n93 = Merge Errors(w17, w16) -> (→"error out 3":errorcluster)
  n94 = case shown="False" "gps" {
    tunnel: w33 -> [_ w222]
    tunnel: ["\u0000" ("format string") w222] -> w32
    frame False {
    }
    frame True {
    }
  }
  n95 = case shown="0, Default" "coarse counter width" {
    tunnel: [u64 1099511625728 ("port") u64 288230376151710720 ("port")] -> w10
    frame 0, Default {
    }
    frame 1 {
    }
  }
  n96 = Increment(x="Counter Setting") -> (x+1=w47:dbl)
  n97 = Divide(x=w51, y="Counter Setting") -> (x/y=w50:dbl)
  n98 = while {
    tunnel: w88 -> [w282]
    tunnel: [w262] -> w59
    tunnel: [w251] -> w81
    shift-right: [w279] -> w63
    shift-left: w8 -> [w280]
    shift-right: [w271] -> _
    shift-left: w58 -> [w278]
    tunnel: "Events" -> [w277]
    shift-right: [w276] -> _
    shift-left: w74 -> [w228]
    shift-right: [w275] -> _
    shift-left: u32 0 ("element") -> [w274]
    shift-right: [w273] -> _
    shift-left: w6 -> [w264]
    shift-right: [w266] -> _
    shift-left: w7 -> [w272]
    tunnel: w12 -> [w258]
    shift-right: [w270] -> _
    shift-left: 0 -> [w245]
    shift-right: [w268] -> _
    shift-left: w29 -> [w267]
    tunnel: w13 -> [_]
    tunnel: w19 -> [w263]
    shift-right: [w259] -> _
    shift-left: w56 -> [w260]
    tunnel: w30 -> [w232]
    tunnel: w51 -> [w256]
    tunnel: w50 -> [w255]
    shift-right: [w250] -> w49
    shift-left: w89 -> [w281]
    tunnel: w47 -> [w249]
    tunnel: w44 -> [w242]
    tunnel: w32 -> [w240]
    tunnel: w29 -> [w239]
    tunnel: "通道数量" -> [w233]
    tunnel: w10 -> [w229]
    shift-right: [w225] -> _
    shift-left: w1 -> [w226]
    stop <- w231 stop-if-true
    n99 = local read "save data"() -> (w244:bool)
    n100 = Dequeue Element(queue=w263) -> (element=w235:string, error out=w262:errorcluster)  [unwired: 2 in, 2 out]
    n101 = case shown="True" w244 {
      tunnel: w282 -> [w295 w303]
      tunnel: w281 -> [w296 w302]
      tunnel: w235 -> [_ w299]
      tunnel: [w296 w298] -> w254
      tunnel: [w295 w297] -> w252
      frame False {
      }
      frame True {
        n102 = Write to Binary File(file (use dialog)=w302, data=w299, error in=w303, 5:FALSE ("prepend array or string size? (T)"), 9:T2."big-endian, network order" ("byte order (0:big-endian, network order)")) -> (refnum out=w298:refnum<file>, error out=w297:errorcluster)  [unwired: 1 in, 1 out]
      }
    }
    n103 = String Length(string=w235) -> (length=w246:i32)
    n104 = case shown="True" TRUE {
      tunnel: w267 -> [w315 w325]
      tunnel: [w315 w326] -> w248
      tunnel: w245 -> [w314 w324]
      tunnel: w246 -> [_ w323]
      tunnel: [w314 w322] -> w247
      tunnel: w242 -> [_ w321]
      tunnel: w239 -> [_ w319]
      tunnel: [FALSE w316] -> w238
      frame False {
      }
      frame True {
        n105 = Get Date/Time In Seconds() -> (seconds since 1Jan1904=w320:timestamp)
        n106 = Subtract(x=w320, y=w325) -> (x-y=w328:dbl)
        n107 = Subtract(x=w320, y=w319) -> (x-y=w318:dbl)
        n108 = Greater Or Equal?(x=w318, y="timeout") -> (x >= y?=w316:bool)
        n109 = Greater Or Equal?(x=w328, y=1.0) -> (x >= y?=w329:bool)
        n110 = case shown="True" w329 {
          tunnel: w328 -> [_ w340]
          tunnel: w320 -> [_ w338]
          tunnel: [w333 w338] -> w326
          tunnel: w325 -> [w333 _]
          tunnel: w324 -> [w332 w335]
          tunnel: w323 -> [w331 _]
          tunnel: [w330 0] -> w322
          tunnel: w321 -> [_ w334]
          frame False {
            n111 = Add(x=w331, y=w332) -> (x+y=w330:i32)
          }
          frame True {
            n112 = Divide(x=w335, y=w334) -> (x/y=w337:dbl)
            n113 = Divide(x=w337, y=w340) -> (x/y=→"rate":dbl)
          }
        }
      }
    }
    n114 = local read "display"() -> (w243:bool)
    n115 = case shown="True" w243 {
      tunnel: w235 -> [_ w294]
      frame False {
      }
      frame True {
        "element" <- w294
      }
    }
    n116 = Unbundle By Name(w262) -> ("status"=w261:bool)
    n117 = case shown="True" "display" {
      tunnel: w264 -> [_ w342]
      tunnel: w228 -> [_ w341]
      frame False {
      }
      frame True {
        "Cal Table" <- w342
        "event" <- w341
      }
    }
    n118 = String Length(string=w235) -> (length=w237:i32)
    n119 = local read "stop"() -> (w230:bool)
    n120 = for {
      N: w237 -> [_]
      tunnel: w235 -> [w291]
      tunnel: [w291] -> w236
      tunnel: [w290] -> w234
      tunnel: w232 -> [w288]
      i -> [w290]
      stop <- w284 stop-if-true
      n121 = Index Array(array=w288) -> (element=w289:string)  [unwired: 1 in]
      n122 = Index Array(array=w288, index=1) -> (element=w286:string)
      n123 = String Subset(string=w291, offset (0)=w290, length (rest)=2 ("length (rest)")) -> (substring=w285:string)
      n124 = Equal?(x=w285, y=w289) -> (x = y?=w292:bool)
      n125 = Equal?(x=w285, y=w286) -> (x = y?=w283:bool)
      n126 = Or(x=w292, y=w283) -> (x .or. y?=w284:bool)
    }
    n127 = case shown="True" "replace dat" {
      tunnel: w254 -> [w305 w311]
      tunnel: [w305 w310] -> w250
      tunnel: w252 -> [w304 w307]
      tunnel: [w304 w306] -> w251
      frame False {
      }
      frame True {
        n128 = Close File(refnum=w311, error in=w307) -> (path=w312:path, error out=w308:errorcluster)
        n129 = Open/Create/Replace File(file path (use dialog)=w312, error in=w308, operation (0:open)=T1."replace or create") -> (refnum out=w310:refnum<file>, error out=w306:errorcluster)  [unwired: 3 in, 1 out]
      }
    }
    n130 = Greater Or Equal?(x=w274, y=w277) -> ()  [unwired: 1 out]
    n131 = Compound Arithmetic op=OR(FALSE ("x"), w261, w238, w230) -> (w231:bool)
    n132 = String Subset(string=w236, offset (0)=w234) -> (substring=w227:string)  [unwired: 1 in]
    n133 = global write "gloabal.vi" "stop"(w231) -> ()
    n134 = while {
      tunnel: w227 -> [w363]
      shift-right: [w433] -> w279
      shift-left: w280 -> [w431]
      shift-right: [w429] -> w271
      shift-left: w278 -> [w430]
      shift-right: [w426] -> w276
      shift-left: w228 -> [w425]
      tunnel: [w424] -> w275
      tunnel: w274 -> [w423]
      shift-right: [w421] -> w273
      shift-left: w264 -> [w422]
      tunnel: w258 -> [w419]
      shift-right: [w418] -> w266
      shift-left: w272 -> [w388]
      shift-right: [w415] -> w259
      shift-left: w260 -> [w416]
      tunnel: w227 -> [w382]
      tunnel: w256 -> [w395]
      tunnel: w255 -> [w394]
      tunnel: w249 -> [w387]
      tunnel: w240 -> [w377]
      tunnel: w233 -> [w365]
      tunnel: w232 -> [w364]
      tunnel: w229 -> [w360]
      tunnel: w227 -> [w350]
      shift-right: [w352] -> w225
      shift-left: w226 -> [w354]
      i -> [w434]
      stop <- w390 stop-if-true
      (unwired) 10 ("length (rest)")
      (unwired) u64 8323072 ("port")
      (unwired) i16 -16 ("y")
      n135 = Multiply(x=w434, y=16 ("length (rest)")) -> (x*y=w355:i32)
      n136 = local read "display"() -> (w417:bool)
      n137 = Add(x=w355, y=8 ("length (rest)")) -> (x+y=w407:i32)
      n138 = Add(x=w355, y=7 ("length (rest)")) -> (x+y=w384:i32)
      n139 = Add(x=w355, y=3 ("length (rest)")) -> (x+y=w357:i32)
      n140 = Add(x=w355, y=0 ("length (rest)")) -> (x+y=w393:i32)
      n141 = String Subset(string=w363, offset (0)=0, length (rest)=2 ("length (rest)")) -> (substring=w366:string)
      "name (unnamed)" <- w366
      n142 = String Subset(string=w363, offset (0)=w393, length (rest)=16 ("y")) -> (substring=w391:string)
      n143 = String Subset(string=w363, offset (0)=w393, length (rest)=8 ("length (rest)")) -> (substring=w375:string)
      n144 = String Subset(string=w382, offset (0)=w407, length (rest)=8 ("length (rest)")) -> (substring=w372:string)
      n145 = String Subset(string=w382, offset (0)=w384, length (rest)=4 ("length (rest)")) -> (substring=w371:string)
      n146 = Search 1D Array(1D array=w364, element=w366) -> (index of element=w367:i32)  [unwired: 1 in]
      n147 = case shown="True" w417 {
        tunnel: w431 -> [_ w480]
        frame False {
        }
        frame True {
          n148 = Index Array(array=w480, index (col)="channel for cal") -> (element=→"cal":i64[])  [unwired: 1 in]
        }
      }
      n149 = String Subset(string=w350, offset (0)=w357, length (rest)=4 ("length (rest)")) -> (substring=w348:string)
      n150 = String Length(string=w391) -> (length=w428:i32)
      n151 = Less?(x=w428, y=16) -> (x < y?=w390:bool)
      n152 = String Subset(string=w375, length (rest)=1 ("length (rest)")) -> (substring=w412:string)  [unwired: 1 in]
      n153 = String Subset(string=w375, offset (0)=7, length (rest)=1 ("length (rest)")) -> (substring=w396:string)
      n154 = Multiply(x=w367, y=w365) -> (x*y=w361:i32)
      n155 = Not Equal?(x="", y=w348) -> (x != y?=w349:bool)
      n156 = String Subset(string=w375, offset (0)=2, length (rest)=1 ("length (rest)")) -> (substring=w373:string)
      n157 = Equal?(x=w412, y="Z" ("format string")) -> (x = y?=w398:bool)
      n158 = Equal?(x=w396, y=w377) -> (x = y?=w397:bool)
      n159 = String To Byte Array(string=w372) -> (unsigned byte array=w404:u8[])
      n160 = String To Byte Array(string=w371) -> (unsigned byte array=w378:u8[])
      n161 = String To Byte Array(string=w373) -> (unsigned byte array=w436:u8[])
      n162 = for {
        shift-right: [w651] -> w401
        shift-left: "" ("format string") -> [w648]
        tunnel: w436 -> [w652] mode=indexing
        n163 = Number To Hexadecimal String(2:w652) -> (0:w644:string)  [unwired: 1 in]
        n164 = String Length(string=w644) -> (length=w650:i32)
        n165 = Equal?(x=w650, y=2) -> (x = y?=w647:bool)
        n166 = Concatenate Strings("0" ("format string"), w644) -> (w646:string)
        n167 = Select(t=w644, s=w647, f=w646) -> (s? t:f=w643:string)
        n168 = Concatenate Strings(w648, w643) -> (w651:string)
      }
      n169 = for {
        shift-right: [w476] -> w402
        shift-left: "" ("format string") -> [w468]
        tunnel: w404 -> [w477] mode=indexing
        n170 = Number To Hexadecimal String(2:w477) -> (0:w470:string)  [unwired: 1 in]
        n171 = String Length(string=w470) -> (length=w475:i32)
        n172 = Concatenate Strings("0" ("format string"), w470) -> (w472:string)
        n173 = Equal?(x=w475, y=2) -> (x = y?=w473:bool)
        n174 = Select(t=w470, s=w473, f=w472) -> (s? t:f=w469:string)
        n175 = Concatenate Strings(w468, w469) -> (w476:string)
      }
      n176 = for {
        shift-right: [w466] -> w381
        shift-left: "" ("format string") -> [w458]
        tunnel: w378 -> [w467] mode=indexing
        n177 = Number To Hexadecimal String(2:w467) -> (0:w460:string)  [unwired: 1 in]
        n178 = String Length(string=w460) -> (length=w465:i32)
        n179 = Concatenate Strings("0" ("format string"), w460) -> (w462:string)
        n180 = Equal?(x=w465, y=2) -> (x = y?=w463:bool)
        n181 = Select(t=w460, s=w463, f=w462) -> (s? t:f=w459:string)
        n182 = Concatenate Strings(w458, w459) -> (w466:string)
      }
      n183 = Not(x=w390) -> (.not. x?=w389:bool)
      n184 = Compound Arithmetic op=AND(w398, w397, w389) -> (w410:bool)
      n185 = Hexadecimal String To Number(string=w401, default (0uL)=u64 0 ("default (0 U32)")) -> (number=w432:u64)  [unwired: 1 in, 1 out]
      n186 = Hexadecimal String To Number(string=w402, default (0uL)=u64 0 ("default (0 U32)")) -> (number=w370:u64)  [unwired: 1 in, 1 out]
      n187 = Hexadecimal String To Number(string=w381, default (0uL)=u64 0 ("default (0 U32)")) -> (number=w359:u64)  [unwired: 1 in, 1 out]
      n188 = And(x=w432, y=u64 127 ("port")) -> (x .and. y?=w362:u64)
      "channel number" <- w362
      n189 = Add(x=w361, y=w362) -> (x+y=w353:u64)
      n190 = case shown="True" w349 {
        tunnel: w354 -> [w438 w444]
        tunnel: w353 -> [_ w442]
        tunnel: [w438 w441] -> w352
        tunnel: w348 -> [_ w440]
        frame False {
        }
        frame True {
          n191 = String To Byte Array(string=w440) -> (unsigned byte array=w445:u8[])
          n192 = for {
            shift-right: [w456] -> w439
            shift-left: "" ("format string") -> [w448]
            tunnel: w445 -> [w457] mode=indexing
            n193 = Number To Hexadecimal String(2:w457) -> (0:w450:string)  [unwired: 1 in]
            n194 = String Length(string=w450) -> (length=w455:i32)
            n195 = Concatenate Strings("0" ("format string"), w450) -> (w452:string)
            n196 = Equal?(x=w455, y=2) -> (x = y?=w453:bool)
            n197 = Select(t=w450, s=w453, f=w452) -> (s? t:f=w449:string)
            n198 = Concatenate Strings(w448, w449) -> (w456:string)
          }
          n199 = Hexadecimal String To Number(string=w439, default (0uL)=u64 0 ("default (0 U32)")) -> (number=w443:u64)  [unwired: 1 in, 1 out]
          n200 = Replace Array Subset(array=w444, new element=w443, index=w442) -> (w441:u32[])
        }
      }
      n201 = case shown="True" w410 {
        tunnel: w370 -> [_ w489]
        tunnel: w423 -> [w484 w504]
        tunnel: w431 -> [w487 w513]
        tunnel: [w487 w512] -> w433
        tunnel: [w486 w509] -> w429
        tunnel: w430 -> [w486 w508]
        tunnel: w353 -> [_ w494]
        tunnel: w425 -> [w485 w507]
        tunnel: [w485 w506] -> w426
        tunnel: [w484 w505] -> w424
        tunnel: w422 -> [w483 w503]
        tunnel: [w483 w502] -> w421
        tunnel: w388 -> [w482 w500]
        tunnel: [w482 w499] -> w418
        tunnel: w419 -> [_ w498]
        tunnel: w416 -> [w481 w496]
        tunnel: [w481 w495] -> w415
        tunnel: w395 -> [_ w493]
        tunnel: w394 -> [_ w492]
        tunnel: w387 -> [_ w491]
        tunnel: w359 -> [_ w490]
        tunnel: w360 -> [_ w488]
        frame False {
          (unwired) FALSE
        }
        frame True {
          n202 = Index Array(array=w503, index=w494) -> (element=w501:u32)
          n203 = Greater?(x=w501, y=w491) -> (0:w497:bool)
          n204 = And(x=w489, y=u64 1023 ("port")) -> (x .and. y?=w510:u64)
          n205 = case shown="True" w497 {
            tunnel: w513 -> [w529 w608]
            tunnel: [w528 w608] -> w512
            tunnel: w510 -> [w520 w566]
            tunnel: [w527 w598] -> w509
            tunnel: w508 -> [w527 w615]
            tunnel: w504 -> [w525 _]
            tunnel: w494 -> [w523 w596]
            tunnel: w507 -> [w526 w614]
            tunnel: [w526 w613] -> w506
            tunnel: [w525 w611] -> w505
            tunnel: w501 -> [w521 _]
            tunnel: w503 -> [w524 w610]
            tunnel: [w522 w610] -> w502
            tunnel: w501 -> [w518 _]
            tunnel: w491 -> [w515 _]
            tunnel: w500 -> [w517 w600]
            tunnel: [w516 w600] -> w499
            tunnel: w498 -> [_ w599]
            tunnel: w496 -> [w514 w593]
            tunnel: [w514 w592] -> w495
            tunnel: w494 -> [_ w589]
            tunnel: w493 -> [_ w587]
            tunnel: w492 -> [_ w588]
            tunnel: w490 -> [_ w582]
            tunnel: w490 -> [_ w571]
            tunnel: w489 -> [_ w565]
            tunnel: w488 -> [_ w563]
            frame False {
              n206 = Equal?(x=w518, y=w515) -> (x = y?=w519:bool)
              n207 = case shown="True" w519 {
                tunnel: w529 -> [w540 w546]
                tunnel: [w538 w546] -> w528
                tunnel: w524 -> [w536 w544]
                tunnel: w523 -> [w535 w541]
                tunnel: [w533 w543] -> w522
                tunnel: w521 -> [w532 w542]
                tunnel: w520 -> [w531 _]
                tunnel: w517 -> [w530 w548]
                tunnel: [w530 w547] -> w516
                frame False {
                  n208 = Index Array(array=w540, index (row)=w531, index (col)=w535) -> (element=w539:i64)
                  n209 = Increment(x=w539) -> (x+1=w537:i64)
                  n210 = Replace Array Subset(array=w540, new element=w537, index (row)=w531, index (col)=w535) -> (w538:i64[][])
                  n211 = Increment(x=w532) -> (x+1=w534:u32)
                  n212 = Replace Array Subset(array=w536, new element=w534, index=w535) -> (w533:u32[])
                  "Calibration Counter" <- w532
                }
                frame True {
                  n213 = for {
                    N: 2048 -> [_]
                    tunnel: w546 -> [w558]
                    tunnel: w541 -> [w551]
                    shift-right: [w553] -> w547
                    shift-left: w548 -> [w554]
                    i -> [w550]
                    n214 = Array Subset(array=w558, index (row)=0 ("索引"), length (row)=w550, index (col)=w551, length (col)=1 ("长度")) -> (w555:i64[][])
                    n215 = Add Array Elements(numeric array=w555) -> (sum=w552:i64)
                    n216 = Replace Array Subset(array=w554, new element=w552, index (row)=w550, index (col)=w551) -> (w553:u32[][])
                  }
                  n217 = Increment(x=w542) -> (x+1=w545:u32)
                  n218 = Replace Array Subset(array=w544, new element=w545, index=w541) -> (w543:u32[])
                }
              }
            }
            frame True {
              (unwired) 0.0 ("x")
              w605 = 0 ("索引 (行)")
              w607 = 1 ("长度")
              # "正式取数"
              n219 = And(x=w571, y=u64 126976 ("port")) -> (x .and. y?=w579:u64)
              n220 = And(x=w582, y=u64 4032 ("port")) -> (x .and. y?=w585:u64)
              n221 = Logical Shift(y=i16 -6, x=w585) -> (x << y=w567:u64)
              n222 = Logical Shift(y=i16 -12, x=w579) -> (x << y=w578:u64)
              n223 = And(x=w571, y=u64 63 ("port")) -> (x .and. y?=w559:u64)
              n224 = And(x=w565, y=w563) -> (x .and. y?=w564:u64)
              "fine 4" <- w564
              n225 = Multiply(x=u64 3600, y=w578) -> (x*y=w574:u64)
              n226 = Multiply(x=u64 60, y=w567) -> (x*y=w575:u64)
              n227 = Logical Shift(y=i16 -10, x=w564) -> (x << y=w561:u64)
              "coarse" <- w561
              n228 = Add(x=w575, y=w574) -> (x+y=w573:u64)
              n229 = Add(x=w573, y=w559) -> (x+y=w562:u64)
              "second stamp" <- w562
              n230 = Add(x=w561, y=w562) -> (x+y=w560:u64)
              n231 = Equal?(x=w589, y=u32 2) -> (x = y?=w591:bool)
              n232 = case shown="True" w591 {
                tunnel: w593 -> [w620 w623]
                tunnel: w560 -> [_ w622]
                tunnel: [w620 w621] -> w592
                frame False {
                }
                frame True {
                  n233 = Build Array (concatenate)(w623, w622) -> (w621:u64[])
                }
              }
              "cal 2" <- w592
              n234 = case shown="True" TRUE {
                tunnel: [w630 w638] -> w617
                tunnel: w608 -> [_ _]
                tunnel: w596 -> [w635 w636]
                tunnel: w566 -> [w633 w641]
                tunnel: w600 -> [w634 w642]
                frame False {
                  w629 = 0 ("index (row)")
                  w632 = 1 ("长度")
                  n235 = Decrement(x=w635) -> (x-1=w628:u64)
                  n236 = Array Subset(array=w634, index (row)=w633, length (row)=w632, index (col)=w628, length (col)=w632) -> (w631:u32[][])
                  n237 = Index Array(array=w631, index (row)=w629, index (col)=w629) -> (element=w630:u32)
                }
                frame True {
                  w637 = 0 ("index (row)")
                  w640 = 1 ("长度")
                  n238 = Array Subset(array=w642, index (row)=w641, length (row)=w640, index (col)=w636, length (col)=w640) -> (w639:u32[][])
                  n239 = Index Array(array=w639, index (row)=w637, index (col)=w637) -> (element=w638:u32)
                }
              }
              n240 = Multiply(x=w560, y=w587) -> (x*y=w570:dbl)
              n241 = Index Array(array=w614, index=w596) -> (element=w611:u32)
              n242 = Array Subset(array=w608, index (row)=w566, length (row)=w607, index (col)=w596, length (col)=w607) -> (w606:i64[][])
              n243 = Index Array(array=w606, index (row)=w605, index (col)=w605) -> (element=w604:i64)
              n244 = Divide(x=w604, y=u32 2) -> (x/y=w609:dbl)
              n245 = Increment(x=w611) -> (x+1=w612:u32)
              n246 = Add(x=w617, y=w609) -> (x+y=w616:dbl)
              n247 = Add(x=w570, y=0.0) -> (x+y=w569:dbl)
              n248 = Multiply(x=w616, y=w588) -> (x*y=w602:dbl)
              n249 = Subtract(x=w587, y=w602) -> (x-y=w586:dbl)
              n250 = Add(x=w586, y=w569) -> (x+y=w603:dbl)
              n251 = Replace Array Subset(array=w614, new element=w612, index=w596) -> (w613:u32[])
              n252 = Replace Array Subset(array=w615, new element=w603, index=w596) -> (w597:dbl[])
              n253 = case shown="True" "save data" {
                tunnel: w599 -> [_ w627]
                tunnel: w597 -> [_ w625]
                frame False {
                }
                frame True {
                  n254 = call-poly <vilib>:"Write Delimited Spreadsheet.vi"("file path (dialog if empty)"=w627, "1D data"=w625, "append to file? (new file:F)"="append csv", "delimiter (\\t)"="," ("delimiter (\\t)")) -> ()  [unwired: 10 in, 2 out]
                }
              }
              n255 = Replace Array Subset(array=w597, new element=0.0 ("new element/subarray"), index=w596) -> (w598:dbl[])
              "fine" <- w566
            }
          }
        }
      }
      n256 = Decimate 1D Array(w352) -> (→"pmt trigger rate":u32[])  [unwired: 1 out]
    }
    n257 = case shown="True" "RST" {
      tunnel: w247 -> [w344 _]
      tunnel: [w344 0] -> w270
      tunnel: [w343 w345] -> w268
      tunnel: w248 -> [w343 _]
      frame False {
      }
      frame True {
        n258 = Get Date/Time In Seconds() -> (seconds since 1Jan1904=w345:timestamp)
      }
    }
  }
  "error out 2" <- w59
  n259 = Close File(refnum=w49, error in=w81) -> (error out=→"error out":errorcluster)  [unwired: 1 out]
  n260 = call-poly <vilib>:"Write Delimited Spreadsheet.vi"("file path (dialog if empty)"=w62, "2D data"=w63, "append to file? (new file:F)"=FALSE, "transpose? (no:F)"=TRUE, "delimiter (\\t)"="," ("delimiter (\\t)")) -> ()  [unwired: 9 in, 2 out]
